vi "setDnsResolver.vi"(8 "error":errorcluster, 9 "resolver":string, 10 "priority":i32, 11 "connection ID":refnum<k5>) -> (0 "error out":errorcluster, 3 "connection ID out":refnum<k5>)   [LabVIEW 2016, in "sen_api.lvlib"]
doc: "Sets the DNS resolver."
uses:
  sen_api.lvlib
panel:
  out "jsonRespIn":string
  out "JSON-response":string="{\"jsonrpc\":\"2.0\",\"method\":\"\",\"params\":[5,1.245,true,\"name\"],\"id\":\"1\"}"
  out "JSON request":string
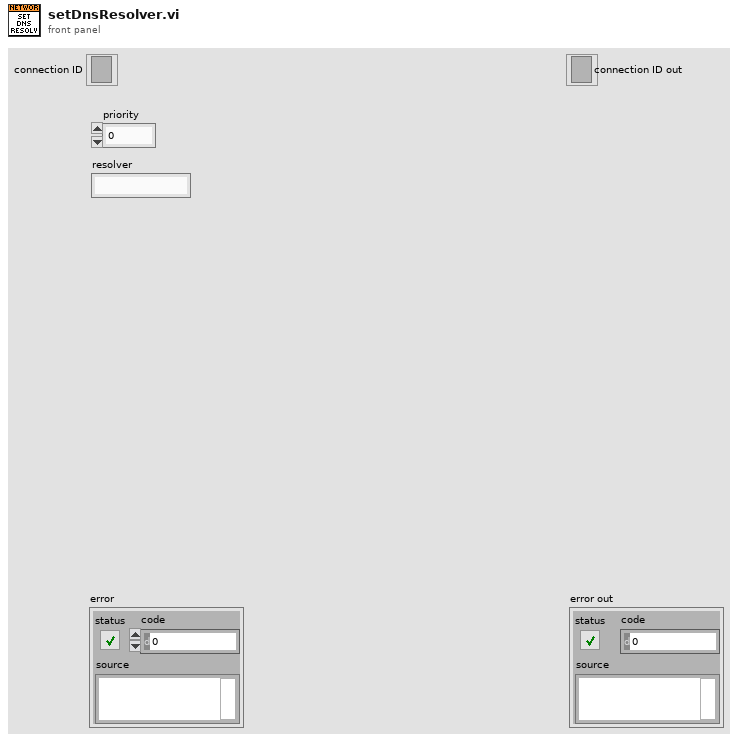
[diagram p1: front panel]
types:
  T1 = cluster{"jsonrpc":string, "method":string, "params":string[], "id":string, "api":i32, "pid":string}
  T2 = enum16{"Standard", "Buffered", "CRLF", "Immediate"}
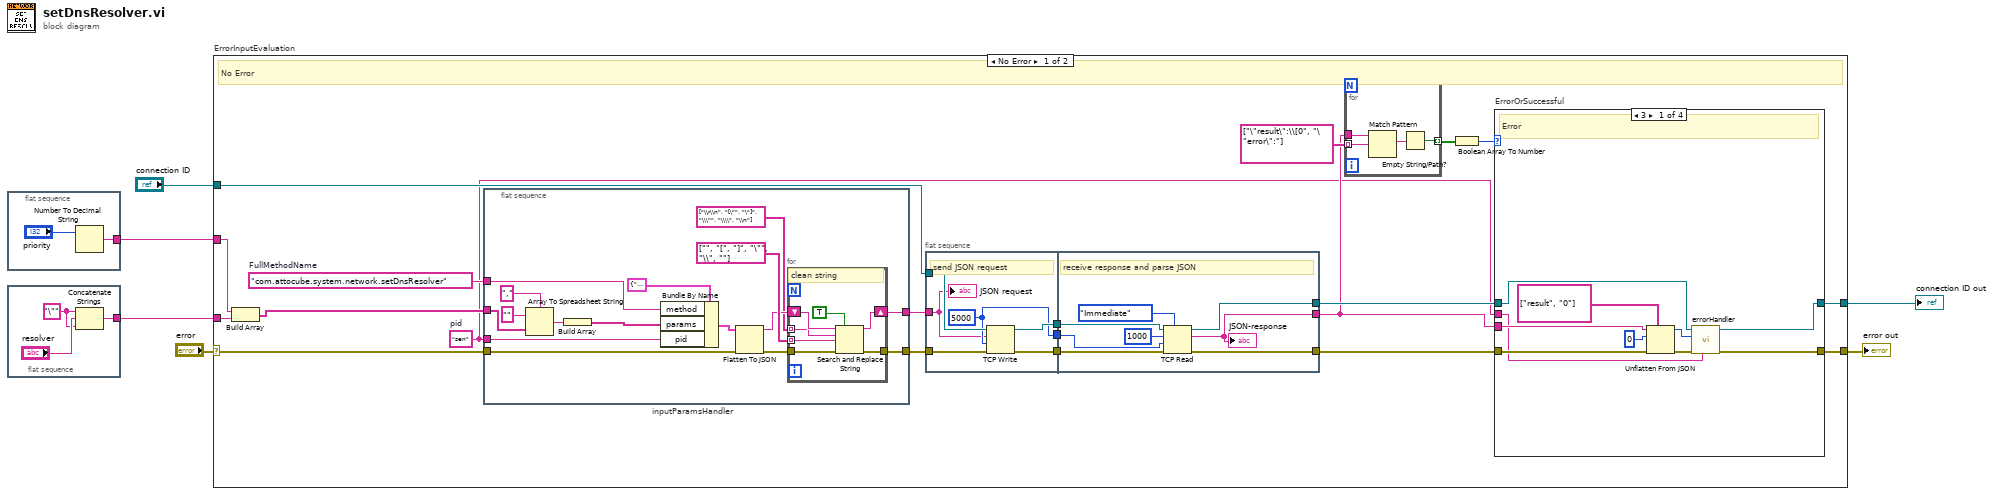
[diagram p0: block diagram]
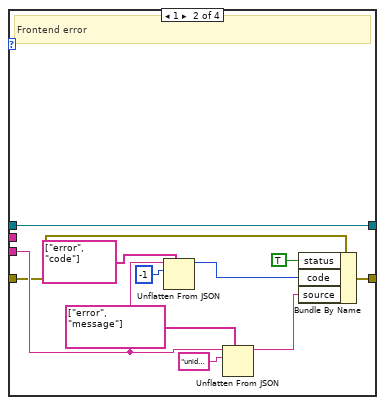
[diagram p2: hidden frame]
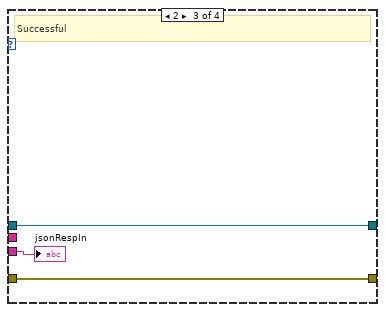
[diagram p3: hidden frame]
diagram:
  n1 = flat-sequence "in_integer" {
    tunnel: [w7] -> w2
    frame #0 {
      n2 = Number To Decimal String(number="priority") -> (decimal integer string=w7:string)  [unwired: 1 in]
    }
  }
  n3 = flat-sequence "in_string" {
    tunnel: [w10] -> w1
    frame #0 {
      w9 = "\"" ("string")
      n4 = Concatenate Strings(w9, "resolver", w9) -> (w10:string)
    }
  }
  n5 = case "ErrorInputEvaluation" shown="No Error" "error" {
    selector: "error" -> [w18 w99]
    tunnel: "connection ID" -> [w28 w100]
    tunnel: [w20 w99] -> w5
    tunnel: [w21 w100] -> w4
    tunnel: w2 -> [w13 _]
    tunnel: w1 -> [w12 _]
    frame No Error {
      w14 = "sen"  # pid
      w19 = "com.attocube.system.network.setDnsResolver"  # FullMethodName
      # "No Error"
      n6 = Build Array ("ParametersArrayString")(w13, w12) -> (w17:string[])
      n7 = flat-sequence "inputParamsHandler" {
        tunnel: [w35] -> w16
        tunnel: w17 -> [w42]
        tunnel: w18 -> [w40]
        tunnel: [w37] -> w15
        tunnel: w19 -> [w43]
        tunnel: w14 -> [w32]
        frame #0 {
          n8 = Array To Spreadsheet String(delimiter (Tab)=",", array=w42, 3:"" ("format string")) -> (spreadsheet string=w45:string)
          n9 = Build Array "Build Array"(w45) -> (w41:string[])
          n10 = Bundle By Name(cluster=T1 {"jsonrpc"="2.0", "method"="com.attocube.amc.res.setRESReadOutFreq", "params"=[], "id"="1", "api"=2, "pid"=""}, "method"=w43, "params"=w41, "pid"=w32) -> (w44:T1)
          n11 = Flatten To JSON(anything=w44, error in (no error)=w40) -> (JSON string=w36:string, 11:w38:errorcluster)  [unwired: 1 in]
          n12 = for {
            tunnel: string[] ["\\r\\n", "[\"", "\"]", "\\\"", "\\\\", "\\n"] ("search string") -> [w51] mode=indexing
            tunnel: string[] ["", "[", "]", "\"", "\\", ""] ("replace string (\"\")") -> [w50] mode=indexing
            shift-right: [w53] -> w35
            shift-left: w36 -> [w52]
            tunnel: w38 -> [w49]
            tunnel: [w48] -> w37
            # "clean string"
            n13 = Search and Replace String(replace all?=TRUE ("replace all? (F)"), input string=w52, search string=w51, replace string=w50, error in=w49) -> (result string=w53:string, error out=w48:errorcluster)  [unwired: 3 in, 2 out]
          }
        }
      }
      n14 = flat-sequence {
        tunnel: w28 -> [w90]
        tunnel: [w88] -> w31
        tunnel: [w89] -> w30
        tunnel: w15 -> [w85]
        tunnel: [w87] -> w29
        tunnel: w16 -> [w86]
        tunnel: [w94] -> w24
        tunnel: w31 -> [w96]
        tunnel: w30 -> [w95]
        tunnel: [w92] -> w23
        tunnel: w29 -> [w93]
        tunnel: [w91] -> w22
        frame #0 {
          w87 = 5000 ("timeout ms (25000)")
          # "send JSON request"
          n15 = TCP Write(connection ID=w90, data in=w86, error in (no error)=w85, 9:w87) -> (connection ID out=w88:refnum<k5>, error out=w89:errorcluster)  [unwired: 1 out]
          "JSON request" <- w86
        }
        frame #1 {
          # "receive response and parse JSON"
          n16 = TCP Read(connection ID=w96, bytes to read=1000, error in (no error)=w95, 7:T2."Immediate" ("mode (standard)"), 9:w93) -> (connection ID out=w94:refnum<k5>, data out=w91:string, error out=w92:errorcluster)
          "JSON-response" <- w91
        }
      }
      n17 = for {
        tunnel: string[] ["\"result\":\\[0", "\"error\":"] ("path") -> [w57] mode=indexing
        tunnel: [w55] -> w26 mode=indexing
        tunnel: w22 -> [w58]
        n18 = Match Pattern(string=w58, regular expression=w57) -> (match substring=w56:string)  [unwired: 1 in, 3 out]
        n19 = Empty String/Path?(string/path=w56) -> (empty?=w55:bool)
      }
      n20 = Boolean Array To Number(Boolean array=w26) -> (number=w25:u32)
      n21 = case "ErrorOrSuccessful" shown="3" w25 {
        tunnel: w22 -> [w62 w71 w80 _]
        tunnel: w24 -> [w66 w69 w82 w84]
        tunnel: [w64 w69 w82 w84] -> w21
        tunnel: [w65 w72 w81 w83] -> w20
        tunnel: w23 -> [w68 w70 w81 w83]
        tunnel: w14 -> [w59 _ _ _]
        frame 3 {
          # "Error"
          n22 = Unflatten From JSON(path=string[] ["result", "0"], JSON string=w62, type and defaults=0, error in (no error)=w68) -> (value=w60:i32, error out=w67:errorcluster)  [unwired: 3 in]
          n23 = call "errorHandler.vi"("pid"=w59, "error in"=w67, "errNbr"=w60, "connection ID"=w66) -> ("error out 2"=w65:errorcluster, "connection ID out"=w64:refnum<k5>)  [unwired: 6 in]
        }
        frame 1 {
          # "Frontend error"
          n24 = Unflatten From JSON(path=string[] ["error", "code"], JSON string=w71, type and defaults=-1) -> (value=w78:i32)  [unwired: 4 in, 1 out]
          n25 = Unflatten From JSON(path=string[] ["error", "message"], JSON string=w71, type and defaults="unidentified error") -> (value=w79:string)  [unwired: 4 in, 1 out]
          n26 = Bundle By Name(cluster=w70, "status"=TRUE, "code"=w78, "source"=w79) -> (w72:errorcluster)
        }
        frame 2 {
          # "Successful"
          "jsonRespIn" <- w80
        }
        frame Default {
          # "NoResponse"
        }
      }
    }
    frame Error {
      # "Error"
    }
  }
  "error out" <- w5
  "connection ID out" <- w4
